vi "timed.vi"() -> ()   [LabVIEW 2016]
uses:
  <vilib>/Platform/TimedLoop/XDataNode/timing_clust.ctl
  <vilib>/Platform/TimedLoop/XDataNode/nitl_modes.ctl
  <vilib>/Platform/TimedLoop/XDataNode/wakeup.ctl
  <vilib>/platform/TimedLoop/XDataNode/XDataNode.xnode
  <vilib>/Platform/TimedLoop/XDataNode/XDNodeRunTimeDep.lvlib
  <instrlib>/Lake Shore 425/Lake Shore 425.lvlib
panel:
  out "XY Graph":cluster{dbl[], dbl[]}[](graph)
  in  "Y-Axis":i32(ring)=6 items=["Time"=0, "x position"=1, "y position"=2, "z position"=3, "Gaussmeter 1"=4, "Gaussmeter 2"=6, "Gaussmeter 3"=8, "Multimeter"=10, "Temperature 1"=11, "Temperature 2"=12, "Temperature 3"=13, "Temperature 4"=14, "Temperature 5"=15, "Temperature 6"=16, "Temperature 7"=17, "Temperature 8"=18]
  in  "X-Axis":i32(ring)=4 items=["Time"=0, "x position"=1, "y position"=2, "z position"=3, "Gaussmeter 1"=4, "Gaussmeter 2"=6, "Gaussmeter 3"=8, "Multimeter"=10, "Temperature 1"=11, "Temperature 2"=12, "Temperature 3"=13, "Temperature 4"=14, "Temperature 5"=15, "Temperature 6"=16, "Temperature 7"=17, "Temperature 8"=18]
  in  "Period [s]":dbl=1.0
  in  "Seconds":dbl
  in  "Minutes":dbl
  in  "Hours":dbl
  in  "Moving Gaussmeter 3":bool caption="Moving"
  in  "x Gaussmeter 3":dbl caption="x [mm]"
  in  "y Gaussmeter 3":dbl caption="y [mm]"
  in  "z Gaussmeter 3":dbl caption="z [mm]"
  in  "Moving Gaussmeter 2":bool caption="Moving"
  in  "x Gaussmeter 2":dbl caption="x [mm]"
  in  "y Gaussmeter 2":dbl caption="y [mm]"
  in  "z Gaussmeter 2":dbl caption="z [mm]"
  in  "z Gaussmeter 1":dbl caption="z [mm]"
  in  "y Gaussmeter 1":dbl caption="y [mm]"
  in  "x Gaussmeter 1":dbl caption="x [mm]"
  in  "Moving Gaussmeter 1":bool caption="Moving"
  out "Time [s]":dbl
  in  "Stop Button":bool
  out "Output File Name":string
  out "Output File Path":path
  in  "Output Folder Path":path=path "C:/Users/ephenix/Dropbox/Stony Brook Research Team Folder/LabVIEW/VI_Argonne/MegaVIEW_v_0_0_5/test output"
  in  "Switch Gaussmeter 3":bool
  in  "VISA resource name Gaussmeter 3":refnum<visa-resource-name>
  out "Probe Type 3":u16(ring)=40 caption="Probe Type" items=["High Sensitivity"=40, "High Stability"=41, "Ultra-High Sensitivity"=42, "User Programmable Cable / High Sensitivity Probe"=50, "User Programmable Cable / High Stability Probe"=51, "User Programmable Cable / Ultra-High Sensitivity Probe"=52]
  out "Probe Serial Number 3":string caption="Probe Serial Number"
  out "Probe Sensitivity 3":dbl=0.001 caption="Probe Sensitivity" format="%^.3e"
  out "Field\nComp 3":bool caption="Field\nComp"
  out "Field Range  3":u16(ring)=1 caption="Field Range" items=["1 - Lowest"=1, "2"=2, "3"=3, "4 - Highest"=4]
  out "Field Units 3":u16(ring)=1 caption="Field Units" items=["Gauss"=1, "Tesla"=2, "Oersted"=3, "Amp/Meter"=4]
  out "Auto\nRange 3":bool caption="Auto\nRange"
  out "Status Gaussmeter 3":bool caption="Status"
  in  "Switch Gaussmeter 2":bool
  in  "VISA resource name Gaussmeter 2":refnum<visa-resource-name>
  out "Probe Type 2":u16(ring)=40 caption="Probe Type" items=["High Sensitivity"=40, "High Stability"=41, "Ultra-High Sensitivity"=42, "User Programmable Cable / High Sensitivity Probe"=50, "User Programmable Cable / High Stability Probe"=51, "User Programmable Cable / Ultra-High Sensitivity Probe"=52]
  out "Probe Serial Number 2":string caption="Probe Serial Number"
  out "Probe Sensitivity 2":dbl=0.001 caption="Probe Sensitivity" format="%^.3e"
  out "Field\nComp 2":bool caption="Field\nComp"
  out "Field Range  2":u16(ring)=1 caption="Field Range" items=["1 - Lowest"=1, "2"=2, "3"=3, "4 - Highest"=4]
  out "Field Units 2":u16(ring)=1 caption="Field Units" items=["Gauss"=1, "Tesla"=2, "Oersted"=3, "Amp/Meter"=4]
  out "Auto\nRange 2":bool caption="Auto\nRange"
  out "Status Gaussmeter 2":bool caption="Status"
  out "Status Gaussmeter 1":bool caption="Status"
  out "Auto\nRange":bool
  out "Field Units":u16(ring)=1 items=["Gauss"=1, "Tesla"=2, "Oersted"=3, "Amp/Meter"=4]
  out "Field Range":u16(ring)=1 items=["1 - Lowest"=1, "2"=2, "3"=3, "4 - Highest"=4]
  out "Field\nComp":bool
  out "Probe Sensitivity":dbl=0.001 format="%^.3e"
  out "Probe Serial Number":string
  out "Probe Type":u16(ring)=40 items=["High Sensitivity"=40, "High Stability"=41, "Ultra-High Sensitivity"=42, "User Programmable Cable / High Sensitivity Probe"=50, "User Programmable Cable / High Stability Probe"=51, "User Programmable Cable / Ultra-High Sensitivity Probe"=52]
  in  "VISA resource name Temperature Monitor":refnum<visa-resource-name>
  in  "VISA resource name Multimeter":refnum<visa-resource-name>
  in  "VISA resource name Gaussmeter 1":refnum<visa-resource-name>
  in  "Switch Temperature Monitor":bool
  in  "Switch Multimeter":bool
  in  "Switch Gaussmeter 1":bool
  out "Waveform Chart Temperature Monitor":dbl(graph)
  out "Waveform Chart Multimeter":dbl(graph)
  out "Waveform Chart Gaussmeter 3":dbl(graph)
  out "Waveform Chart Gaussmeter 2":dbl(graph)
  out "Waveform Chart Gaussmeter 1":dbl(graph)
  # "Gaussmeter 1 (Lake Shore 425)"
  # "Gaussmeter 2 (Lake Shore 425)"
  # "Gaussmeter 3 (Lake Shore 425)"
  # "Multimeter (Agilent 34461A)"
  # "Temperature Monitor (Lake Shore 218)"
  # "XY Graph Axes"
  # "Duration"
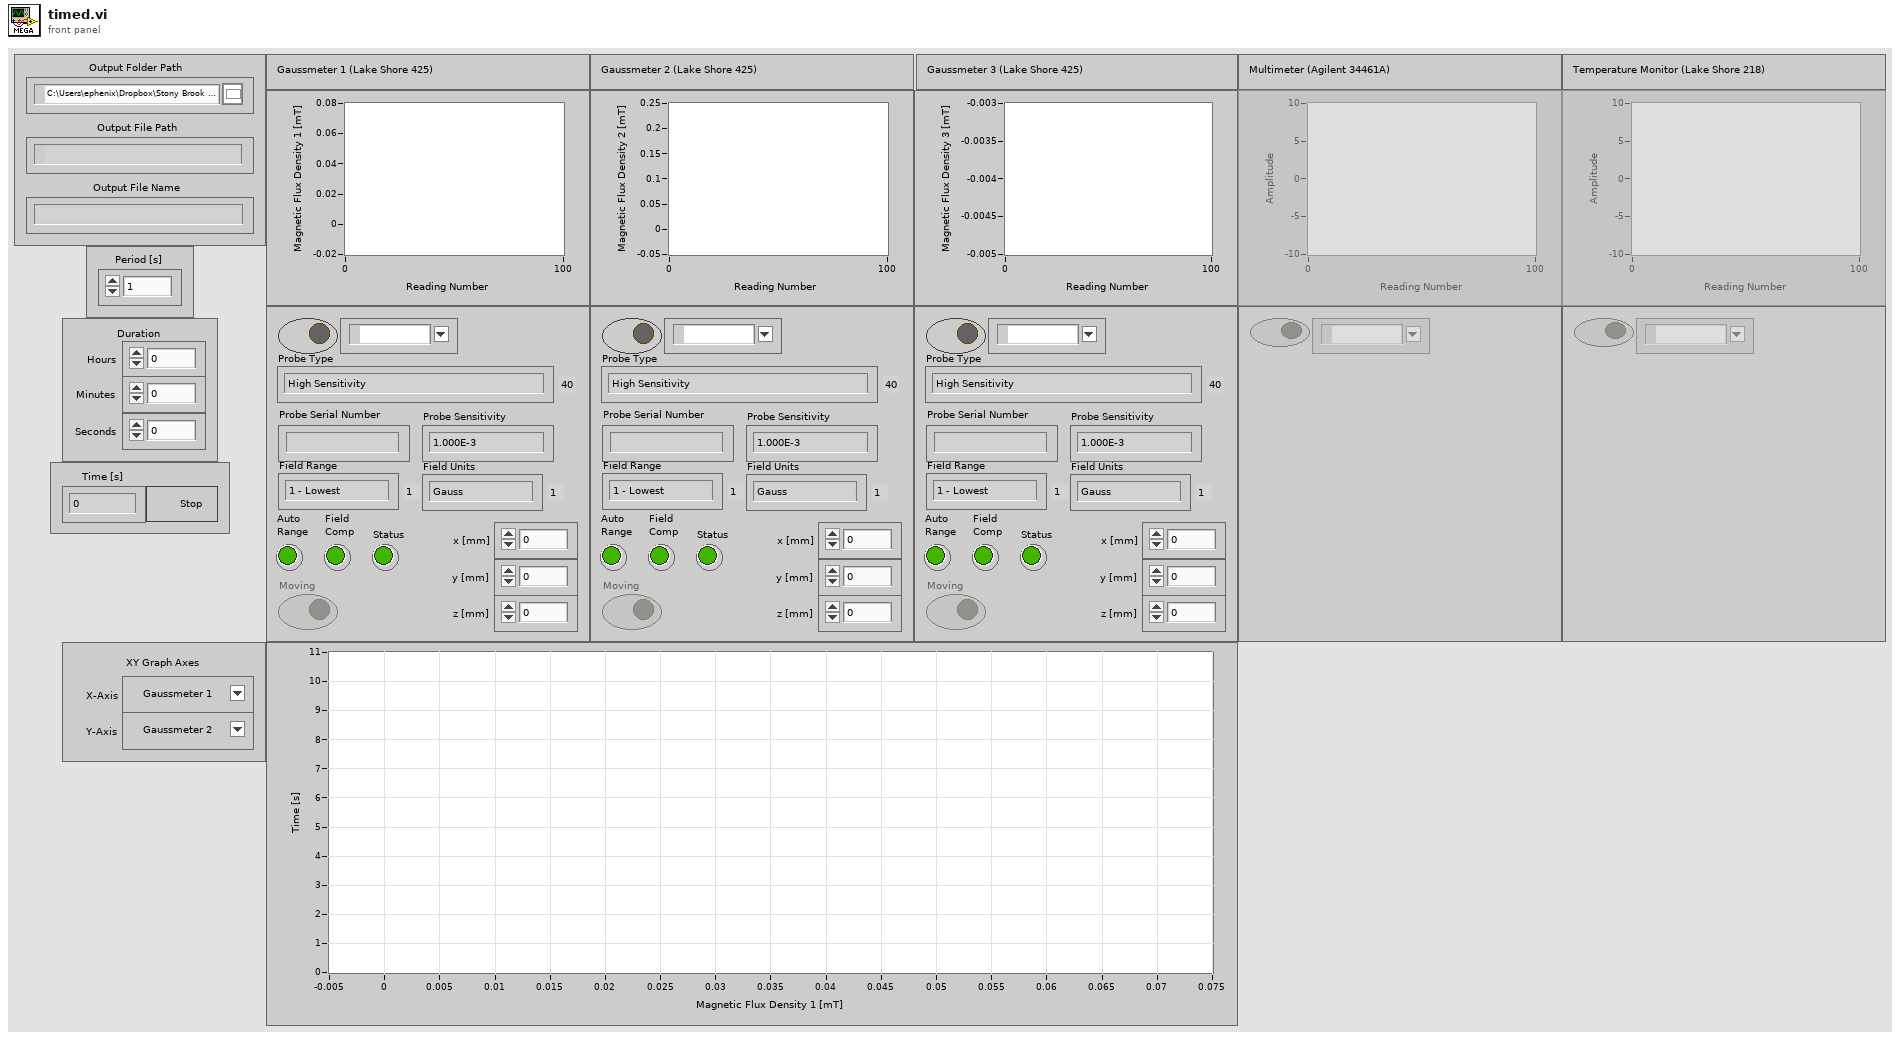
[diagram p1: front panel]
types:
  T1 = cluster{"Gaussmeter VISA resource name out":refnum<visa-resource-name>, "Switch Gaussmeter 1":bool, "Gaussmeter VISA resource name out":refnum<visa-resource-name>, "Switch Gaussmeter 2":bool, "Gaussmeter VISA resource name out":refnum<visa-resource-name>, "Switch Gaussmeter 3":bool}
  T2 = typedef "XDNodeRunTimeDep.lvlib/timing_clust.ctl" = cluster{"Expected End [f-1]":u64, "Actual End [f-1]":u64, "Finished Late? [f-1]":bool, "Expected End [i-1]":u64, "Actual End [i-1]":u64, "Finished Late? [i-1]":bool, "Expected Start [i]":u64, "Actual Start [i]":u64, "Expected Start [f]":u64, "Actual Start [f]":u64, "Source Name":string, "Structure Name":string, "Period":i64, "Deadline":i64, "Offset":i64, "Start":i64, "Priority":i32, "Timeout":i32, "Mode":T3, "Wakeup Reason":T4, "Error":errorcluster, "Source Type":string, "Secondary Source Type":string, "Global End Time":u64, "Global Start Time":u64, "Frame Duration":u64, "Iteration Duration":u64, "Assigned CPU":i32, "I/O Scan Engine Mode":u32}
  T3 = typedef "XDNodeRunTimeDep.lvlib/nitl_modes.ctl" = enum32{"No Change", "Process missed periods, maintain original phase", "Discard missed periods, maintain original phase", "Process missed periods, ignore original phase", "Discard missed periods, ignore original phase"}
  T4 = typedef "XDNodeRunTimeDep.lvlib/wakeup.ctl" = enum32{"Normal", "Aborted", "Asynchronous wakeup", "Timing source error", "Timed loop error", "Timeout"}
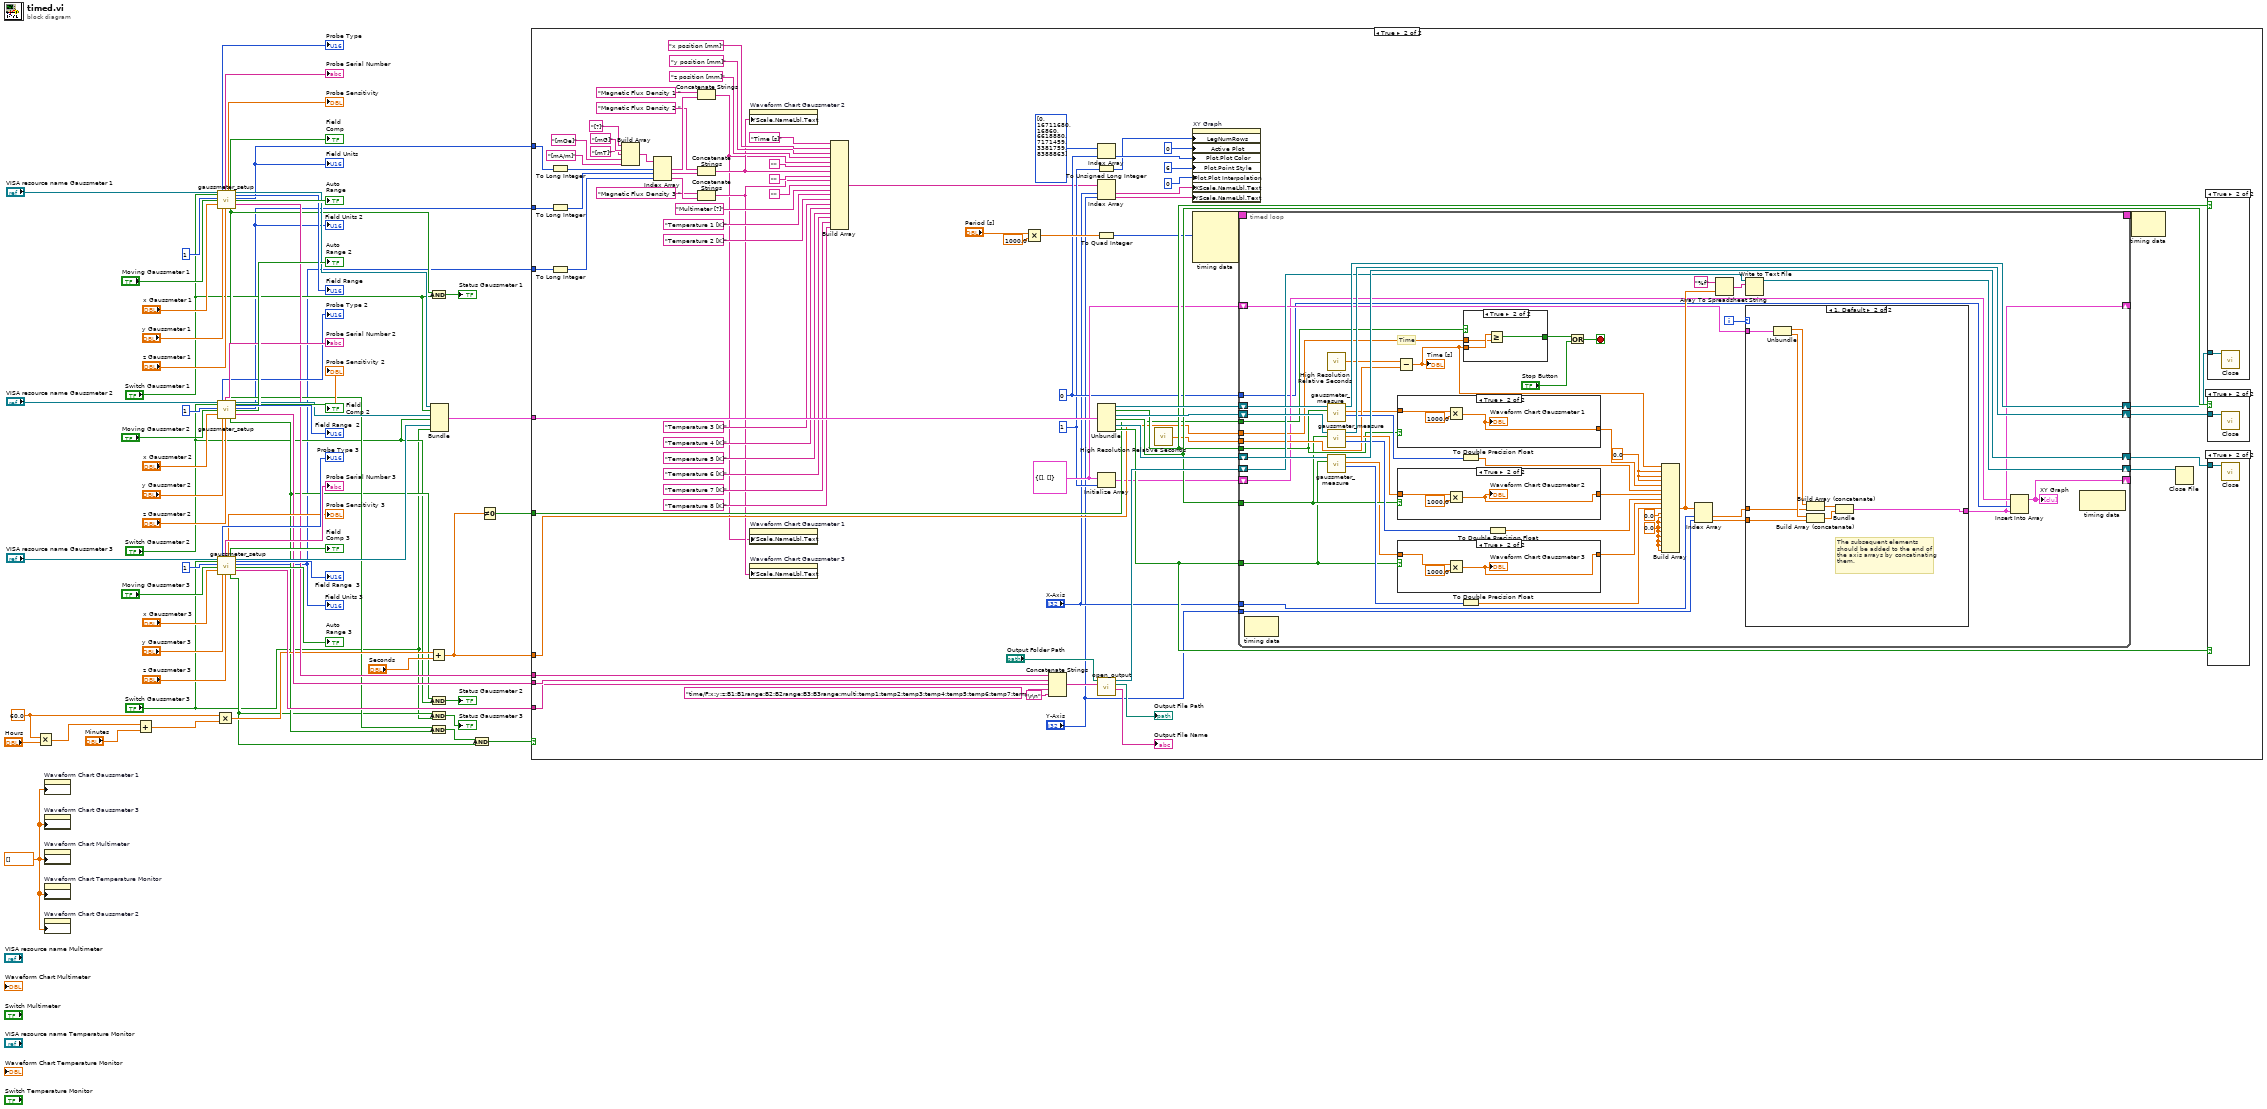
[diagram p0: block diagram]
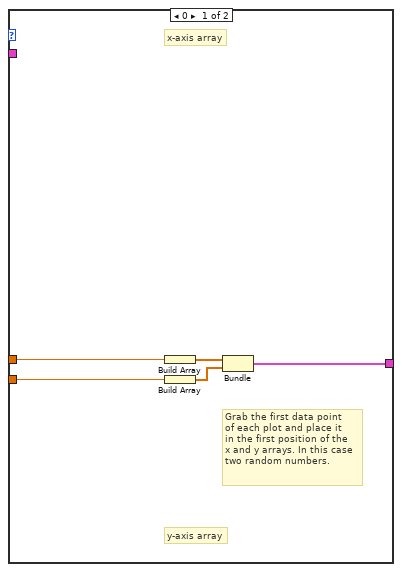
[diagram p6: hidden frame]
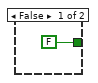
[diagram p10: hidden frame]
diagram:
  w4 = dbl[] [] ("History Data")
  w18 = 60.0
  n1 = Multiply(x=w18, y="Hours") -> (x*y=w21:dbl)
  n2 = property on="Waveform Chart Gaussmeter 1" class="WFChart (strict)"("History Data"=w4) -> ()  [unwired: 2 in, 2 out]
  n3 = property on="Waveform Chart Gaussmeter 3" class="WFChart (strict)"("History Data"=w4) -> ()  [unwired: 2 in, 2 out]
  n4 = property on="Waveform Chart Multimeter" class="WFChart (strict)"("History Data"=w4) -> ()  [unwired: 2 in, 2 out]
  n5 = property on="Waveform Chart Temperature Monitor" class="WFChart (strict)"("History Data"=w4) -> ()  [unwired: 2 in, 2 out]
  n6 = property on="Waveform Chart Gaussmeter 2" class="WFChart (strict)"("History Data"=w4) -> ()  [unwired: 2 in, 2 out]
  n7 = Add(x=w21, y="Minutes") -> (x+y=w19:dbl)
  n8 = Multiply(x=w18, y=w19) -> (x*y=w17:dbl)
  n9 = call "gaussmeter_setup.vi"("VISA resource name Gaussmeter"="VISA resource name Gaussmeter 1", "Switch Gaussmeter"="Switch Gaussmeter 1", "Gaussmeter Number"=u8 1, "Moving Gaussmeter"="Moving Gaussmeter 1", "x Gaussmeter"="x Gaussmeter 1", "y Gaussmeter"="y Gaussmeter 1", "z Gaussmeter"="z Gaussmeter 1") -> ("Probe Type"=→"Probe Type":u16, "Probe Serial Number"=→"Probe Serial Number":string, "Probe Sensitivity"=→"Probe Sensitivity":dbl, "Probe Field\nCompensation On"=→"Field\nComp":bool, "Status Gaussmeter"=w12:bool, "Gaussmeter VISA resource name out"=w44:refnum<visa-resource-name>, "Field Range"=→"Field Range":u16, "Field Units"=w1:u16, "Auto Range On"=→"Auto\nRange":bool, "Text Output"=w38:string)  [unwired: 2 in, 1 out]
  "Field Units" <- w1
  n10 = call "gaussmeter_setup.vi"("VISA resource name Gaussmeter"="VISA resource name Gaussmeter 2", "Switch Gaussmeter"="Switch Gaussmeter 2", "Gaussmeter Number"=u8 1, "Moving Gaussmeter"="Moving Gaussmeter 2", "x Gaussmeter"="x Gaussmeter 2", "y Gaussmeter"="y Gaussmeter 2", "z Gaussmeter"="z Gaussmeter 2") -> ("Probe Type"=→"Probe Type 2":u16, "Probe Serial Number"=→"Probe Serial Number 2":string, "Probe Sensitivity"=→"Probe Sensitivity 2":dbl, "Probe Field\nCompensation On"=→"Field\nComp 2":bool, "Status Gaussmeter"=w9:bool, "Gaussmeter VISA resource name out"=w43:refnum<visa-resource-name>, "Field Range"=→"Field Range  2":u16, "Field Units"=w2:u16, "Auto Range On"=→"Auto\nRange 2":bool, "Text Output"=w37:string)  [unwired: 2 in, 1 out]
  "Field Units 2" <- w2
  n11 = call "gaussmeter_setup.vi"("VISA resource name Gaussmeter"="VISA resource name Gaussmeter 3", "Switch Gaussmeter"="Switch Gaussmeter 3", "Gaussmeter Number"=u8 1, "Moving Gaussmeter"="Moving Gaussmeter 3", "x Gaussmeter"="x Gaussmeter 3", "y Gaussmeter"="y Gaussmeter 3", "z Gaussmeter"="z Gaussmeter 3") -> ("Probe Type"=→"Probe Type 3":u16, "Probe Serial Number"=→"Probe Serial Number 3":string, "Probe Sensitivity"=→"Probe Sensitivity 3":dbl, "Probe Field\nCompensation On"=→"Field\nComp 3":bool, "Status Gaussmeter"=w7:bool, "Gaussmeter VISA resource name out"=w42:refnum<visa-resource-name>, "Field Range"=→"Field Range  3":u16, "Field Units"=w3:u16, "Auto Range On"=→"Auto\nRange 3":bool, "Text Output"=w36:string)  [unwired: 2 in, 1 out]
  "Field Units 3" <- w3
  n12 = And(x=w12, y="Switch Gaussmeter 1") -> (x .and. y?=→"Status Gaussmeter 1":bool)
  n13 = Add(x=w17, y="Seconds") -> (x+y=w14:dbl)
  n14 = And(x=w9, y="Switch Gaussmeter 2") -> (x .and. y?=→"Status Gaussmeter 2":bool)
  n15 = And(x=w7, y="Switch Gaussmeter 3") -> (x .and. y?=→"Status Gaussmeter 3":bool)
  n16 = And(x=w12, y=w9) -> (x .and. y?=w41:bool)
  n17 = Bundle("Gaussmeter VISA resource name out"=w44, "Switch Gaussmeter 1"="Switch Gaussmeter 1", "Gaussmeter VISA resource name out"=w43, "Switch Gaussmeter 2"="Switch Gaussmeter 2", "Gaussmeter VISA resource name out"=w42, "Switch Gaussmeter 3"="Switch Gaussmeter 3") -> (w39:T1)  [unwired: 1 in]
  n18 = And(x=w41, y=w7) -> (x .and. y?=w40:bool)
  n19 = Not Equal To 0?(x=w14) -> (x != 0?=w15:bool)
  n20 = case shown="True" w40 {
    tunnel: w39 -> [_ w147]
    tunnel: w38 -> [_ w139]
    tunnel: w37 -> [_ w138]
    tunnel: w36 -> [_ w137]
    tunnel: w15 -> [_ w125]
    tunnel: w14 -> [_ w124]
    tunnel: w3 -> [_ w79]
    tunnel: w2 -> [_ w78]
    tunnel: w1 -> [_ w77]
    frame False {
    }
    frame True {
      w117 = 0
      w110 = 1 ("dimension size")
      w119 = cluster{dbl[], dbl[]} {[], []}
      n21 = To Long Integer(number=w77) -> (32bit integer=w83:i32)
      n22 = To Long Integer(number=w78) -> (32bit integer=w81:i32)
      n23 = To Long Integer(number=w79) -> (32bit integer=w80:i32)
      n24 = Build Array("[?]", "[mG]", "[mT]", "[mOe]", "[mA/m]") -> (w82:string[])
      n25 = Index Array(array=w82, index #1=w83, index #2=w81, index #3=w80) -> (element #1=w74:string, element #2=w75:string, element #3=w76:string)
      n26 = Concatenate Strings("Magnetic Flux Density 1 ", w74) -> (w68:string)
      n27 = Concatenate Strings("Magnetic Flux Density 2 ", w75) -> (w69:string)
      n28 = Concatenate Strings("Magnetic Flux Density 3 ", w76) -> (w70:string)
      n29 = property on="Waveform Chart Gaussmeter 2" class="WFChart (strict)"("YScale.NameLbl.Text"=w69) -> ()  [unwired: 2 in, 2 out]
      n30 = property on="Waveform Chart Gaussmeter 1" class="WFChart (strict)"("YScale.NameLbl.Text"=w68) -> ()  [unwired: 2 in, 2 out]
      n31 = property on="Waveform Chart Gaussmeter 3" class="WFChart (strict)"("YScale.NameLbl.Text"=w70) -> ()  [unwired: 2 in, 2 out]
      n32 = Build Array("Time [s]", "x position [mm]", "y position [mm]", "z position [mm]", w68, "", w69, "", w70, "", "Multimeter [?]", "Temperature 1 [K]", "Temperature 2 [K]", "Temperature 3 [K]", "Temperature 4 [K]", "Temperature 5 [K]", "Temperature 6 [K]", "Temperature 7 [K]", "Temperature 8 [K]") -> (w103:string[])
      n33 = Multiply(x="Period [s]", y=1000.0) -> (x*y=w120:dbl)
      n34 = Concatenate Strings(w139, w138, w137, "time/F:x:y:z:B1:B1range:B2:B2range:B3:B3range:multi:temp1:temp2:temp3:temp4:temp5:temp6:temp7:temp8", "\r\n") -> (w140:string)
      n35 = To Unsigned Long Integer(number=w110) -> (unsigned 32bit integer=w111:u32)
      n36 = To Quad Integer(1:w120) -> (0:w123:i64)
      n37 = Index Array(array=u32[] [0, 16711680, 16860, 6618880, 7171459, 3381759, 8388863], index=w117) -> (element=w115:u32)
      n38 = Index Array(array=w103, index #1="X-Axis", index #2="Y-Axis") -> (element #1=w102:string, element #2=w101:string)
      n39 = Unbundle(w147) -> ("Gaussmeter VISA resource name out"=w146:refnum<visa-resource-name>, "Switch Gaussmeter 1"=w130:bool, "Gaussmeter VISA resource name out"=w145:refnum<visa-resource-name>, "Switch Gaussmeter 2"=w131:bool, "Gaussmeter VISA resource name out"=w144:refnum<visa-resource-name>, "Switch Gaussmeter 3"=w132:bool)
      n40 = Initialize Array(w119, w110) -> (w118:cluster{dbl[], dbl[]}[])
      n41 = call "open_output.vi"("Output File Header"=w140, "Output Folder Path"="Output Folder Path") -> ("Output File Name"=→"Output File Name":string, "Output File Path"=→"Output File Path":path, "refnum out"=w134:refnum<file>)  [unwired: 7 in]
      n42 = call <vilib>:"High Resolution Relative Seconds.vi"() -> ("relative seconds"=w126:dbl)
      n43 = property on="XY Graph" class="XYGraph (strict)"("LegNumRows"=w111, "Active Plot"=u32 0, "Plot.Plot Color"=w115, "Plot.Point Style"=u8 6, "Plot.Plot Interpolation"=u8 0, "XScale.NameLbl.Text"=w102, "YScale.NameLbl.Text"=w101) -> ()  [unwired: 2 in, 2 out]
      n44 = node-c288(w123) -> (w149:T2)  [unwired: 3 in]
      n45 = timed-loop {
        timing: w149 -> [_]
        timing-out: [_] -> w148
        shift-right: [w194] -> w129
        shift-left: w146 -> [w199]
        tunnel: w130 -> [w170]
        shift-right: [w195] -> w128
        shift-left: w145 -> [w198]
        shift-right: [w196] -> w127
        shift-left: w144 -> [w197]
        tunnel: w131 -> [w169]
        tunnel: w132 -> [w168]
        shift-right: [w184] -> w133
        shift-left: w134 -> [w185]
        tunnel: w126 -> [w179]
        tunnel: w125 -> [w178]
        tunnel: w124 -> [w176]
        tunnel: "X-Axis" -> [w167]
        tunnel: "Y-Axis" -> [w166]
        shift-right: [w158] -> _
        shift-left: w119 -> [w161]
        shift-right: [w157] -> _
        shift-left: w118 -> [w160]
        tunnel: w117 -> [w159]
        i -> [w164]
        stop <- w173 stop-if-true
        w182 = 0.0
        w187 = 0.0
        # "Time"
        n46 = node-c288() -> ()  [unwired: 1 in, 1 out]
        n47 = call <vilib>:"High Resolution Relative Seconds.vi"() -> ("relative seconds"=w180:dbl)
        n48 = call "gaussmeter_measure.vi"("Switch Gaussmeter"=w170, "VISA resource name"=w199) -> ("Field Range"=w192:u16, "Field Reading"=w172:dbl, "VISA resource name out"=w194:refnum<visa-resource-name>)  [unwired: 5 in, 2 out]
        n49 = call "gaussmeter_measure.vi"("Switch Gaussmeter"=w169, "VISA resource name"=w198) -> ("Field Range"=w191:u16, "Field Reading"=w171:dbl, "VISA resource name out"=w195:refnum<visa-resource-name>)  [unwired: 5 in, 2 out]
        n50 = call "gaussmeter_measure.vi"("Switch Gaussmeter"=w168, "VISA resource name"=w197) -> ("Field Range"=w190:u16, "Field Reading"=w154:dbl, "VISA resource name out"=w196:refnum<visa-resource-name>)  [unwired: 5 in, 2 out]
        n51 = Subtract(x=w180, y=w179) -> (x-y=w177:dbl)
        "Time [s]" <- w177
        n52 = case shown="True" w170 {
          tunnel: w172 -> [w221 w223]
          tunnel: [w221 w222] -> w156
          frame False {
          }
          frame True {
            n53 = Multiply(x=w223, y=1000.0) -> (x*y=w222:dbl)
            "Waveform Chart Gaussmeter 1" <- w222
          }
        }
        n54 = case shown="True" w169 {
          tunnel: w171 -> [w217 w219]
          tunnel: [w217 w218] -> w153
          frame False {
          }
          frame True {
            n55 = Multiply(x=w219, y=1000.0) -> (x*y=w218:dbl)
            "Waveform Chart Gaussmeter 2" <- w218
          }
        }
        n56 = case shown="True" w168 {
          tunnel: w154 -> [w213 w215]
          tunnel: [w213 w214] -> w155
          frame False {
          }
          frame True {
            n57 = Multiply(x=w215, y=1000.0) -> (x*y=w214:dbl)
            "Waveform Chart Gaussmeter 3" <- w214
          }
        }
        n58 = To Double Precision Float(number=w192) -> (double precision float=w193:dbl)
        n59 = To Double Precision Float(number=w190) -> (double precision float=w188:dbl)
        n60 = case shown="True" w178 {
          tunnel: w177 -> [_ w228]
          tunnel: w176 -> [_ w227]
          tunnel: [FALSE w226] -> w175
          frame False {
          }
          frame True {
            n61 = Greater Or Equal?(x=w228, y=w227) -> (x >= y?=w226:bool)
          }
        }
        n62 = To Double Precision Float(number=w191) -> (double precision float=w189:dbl)
        n63 = Or(x=w175, y="Stop Button") -> (x .or. y?=w173:bool)
        n64 = Build Array(w177, w187, w187, w187, w156, w193, w153, w189, w155, w188, 0.0, w182, w182, w182, w182, w182, w182, w182, w182) -> (w165:dbl[])
        n65 = Index Array(array=w165, index #1=w167, index #2=w166) -> (element #1=w163:dbl, element #2=w162:dbl)
        n66 = Array To Spreadsheet String(array=w165, 3:"%f" ("format string")) -> (spreadsheet string=w186:string)  [unwired: 1 in]
        n67 = Write to Text File(file (use dialog)=w185, text=w186) -> (refnum out=w184:refnum<file>)  [unwired: 2 in, 2 out]
        n68 = case shown="1, Default" w164 {
          tunnel: [w202 w209] -> w158
          tunnel: w161 -> [_ w205]
          tunnel: w162 -> [w200 w207]
          tunnel: w163 -> [w201 w206]
          frame 0 {
            # "y-axis array"
            # "x-axis array"
            # "Grab the first data point\nof each plot and place it\nin the first position of the \nx and y arrays. In this case\ntwo random numbers."
            n69 = Build Array(w201) -> (w204:dbl[])
            n70 = Build Array(w200) -> (w203:dbl[])
            n71 = Bundle(w204, w203) -> (w202:cluster{dbl[], dbl[]})  [unwired: 1 in]
          }
          frame 1, Default {
            # "The subsequent elements\nshould be added to the end of\nthe axis arrays by concatinating\nthem."
            n72 = Unbundle(w205) -> (w212:dbl[], w208:dbl[])
            n73 = Build Array (concatenate)(w212, w206) -> (w211:dbl[])
            n74 = Build Array (concatenate)(w208, w207) -> (w210:dbl[])
            n75 = Bundle(w211, w210) -> (w209:cluster{dbl[], dbl[]})  [unwired: 1 in]
          }
        }
        n76 = Insert Into Array(array=w160, index=w159, new element=w158) -> (w157:cluster{dbl[], dbl[]}[])
        "XY Graph" <- w157
        n77 = node-c288() -> ()  [unwired: 1 in, 1 out]
      }
      n78 = node-c288(w148) -> ()  [unwired: 1 out]
      n79 = Close File(refnum=w133) -> ()  [unwired: 1 in, 2 out]
      n80 = case shown="True" w130 {
        tunnel: w129 -> [_ w152]
        frame False {
        }
        frame True {
          n81 = call <instrlib>:"Close.vi"("VISA resource name"=w152) -> ()  [unwired: 10 in, 1 out]
        }
      }
      n82 = case shown="True" w131 {
        tunnel: w128 -> [_ w151]
        frame False {
        }
        frame True {
          n83 = call <instrlib>:"Close.vi"("VISA resource name"=w151) -> ()  [unwired: 10 in, 1 out]
        }
      }
      n84 = case shown="True" w132 {
        tunnel: w127 -> [_ w150]
        frame False {
        }
        frame True {
          n85 = call <instrlib>:"Close.vi"("VISA resource name"=w150) -> ()  [unwired: 10 in, 1 out]
        }
      }
    }
  }
